vi "NI VeriStand - Set Loop Type.vi"(8 "error in (no error)":errorcluster, 9 "Use Device Clock (Timed Loops only)":bool, 10 "Loop type":T1, 11 "Device Ref in":T2 format="%.0x") -> (0 "error out":errorcluster, 3 "Device Ref out":T2 format="%.0x")   [LabVIEW 2020, in "Custom Device API.lvlib"]
doc: "Specifies whether the asynchronous custom device uses a While Loop or a Timed Loop. If <B>Loop type</B> is 1 - Timed Loop, you can use the <B>Use Device Clock</B> input to synchronize the loop to the Primary Control Loop's timing source. Do not use this VI on inline custom devices."
uses:
  <vilib>/NI VeriStand/Custom Device API/Custom Device API.lvlib
  <vilib>/NI VeriStand/Custom Device API/Custom Device Item Ref.ctl
  <vilib>/NI VeriStand/Custom Device API/Custom Device Loop Type.ctl
  26443dc4-0133-4b48-92d3-5cb9ea2206ed.vi
  <vilib>/NI VeriStand/Custom Device API/Custom Device Offline Path.vi
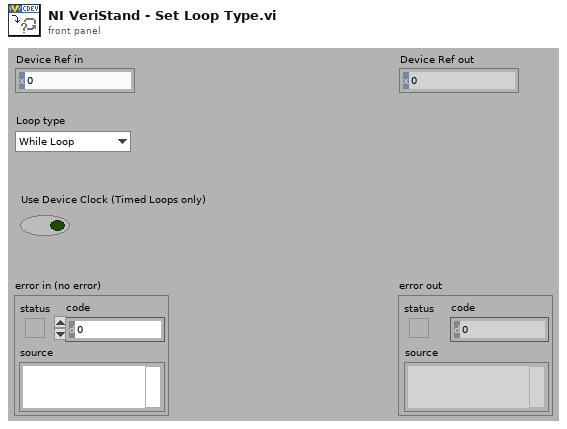
[diagram p1: front panel]
types:
  T1 = typedef "Custom Device API.lvlib/Custom Device Loop Type.ctl" = enum32{"While Loop", "Timed Loop"}
  T2 = typedef "Custom Device API.lvlib/Custom Device Item Ref.ctl" = u64
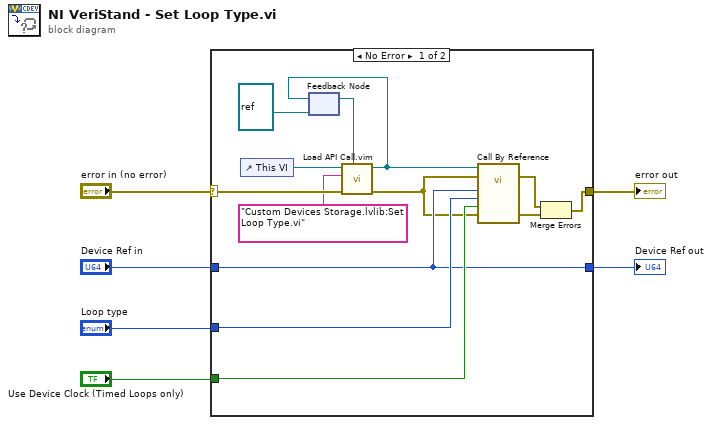
[diagram p0: block diagram]
diagram:
  n1 = case shown="No Error" "error in (no error)" {
    selector: "error in (no error)" -> [w12 w21]
    tunnel: [w18 w21] -> w6
    tunnel: "Device Ref in" -> [w15 w20]
    tunnel: "Loop type" -> [w17 _]
    tunnel: "Use Device Clock (Timed Loops only)" -> [w16 _]
    tunnel: [w15 w20] -> w2
    frame No Error {
      n2 = control-ref of="This VI"() -> (w13:refnum<vi>)
      n3 = feedback #1(refnum<vi> refnum ("type specifier VI Refnum (for type only)")) -> (w14:refnum<vi>)
      n4 = call "Load API Call.vim"("VI reference in"=w14, "error in (no error)"=w12, "VI qualified name"="Custom Devices Storage.lvlib:Set Loop Type.vi", "Caller VI ref"=w13) -> ("error out"=w11:errorcluster, "VI reference"=w10:refnum<vi>)  [unwired: 6 in]
      n5 = feedback-in #1(w10) -> ()
      n6 = call-by-ref "?"(reference=w10, error in=w11, 8:"error in (no error)"=w11, "Use Device Clock (Timed Loops only)"=w16, "Loop type"=w17, "Device Ref in"=w15) -> (error out=w7:errorcluster, 0:"error out"=w19:errorcluster)  [unwired: 6 in, 2 out]
      n7 = Merge Errors(w7, w19) -> (w18:errorcluster)
    }
    frame Error {
    }
  }
  "Device Ref out" <- w2
  "error out" <- w6
